vi "Check number of products.vi"(9 "Product name":string, 11 "Data Cluster":T1) -> (3 "Product Available":bool)   [LabVIEW 2020, in "Stock.lvlib"]
uses:
  Stock.lvlib
  Module Data--cluster.ctl
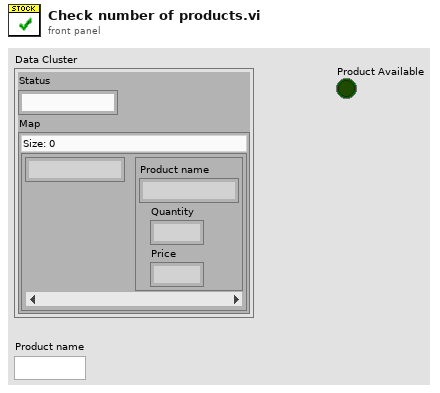
[diagram p1: front panel]
types:
  T1 = typedef "Stock.lvlib/Module Data--cluster.ctl" = cluster{"Status":string, "Map":map{string, cluster{"Product name":string, "Quantity":dbl, "Price":dbl}}}
  T2 = map{string, cluster{"Product name":string, "Quantity":dbl, "Price":dbl}}
  T3 = cluster{"Product name":string, "Quantity":dbl, "Price":dbl}
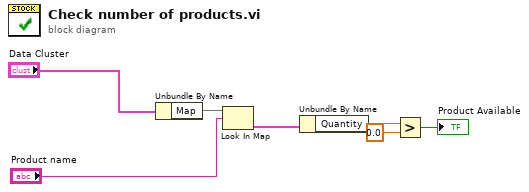
[diagram p0: block diagram]
diagram:
  n1 = Unbundle By Name("Data Cluster") -> ("Map"=w7:T2)
  n2 = Look In Map(map=w7, key="Product name") -> (value=w4:T3)  [unwired: 1 in, 1 out]
  n3 = Unbundle By Name(w4) -> ("Quantity"=w3:dbl)
  n4 = Greater?(x=w3, y=0.0) -> (0:→"Product Available":bool)
